vi "Global_CMD_.vi"() -> ()   [LabVIEW 2016]
panel:
  in  "CMD_Subsystem_DBL":dbl
  in  "CMD_Subsystem_Bool":bool
  # "The Names of the Data items in the Global Variable MUST describe who the Single Writer is\nNaming Convention for Command Globals is:   \n\nCMD_SubSystem_Data Name\nExample:\nCMD_Drive_Mode\nCMD_Hopper_Fire Ball"
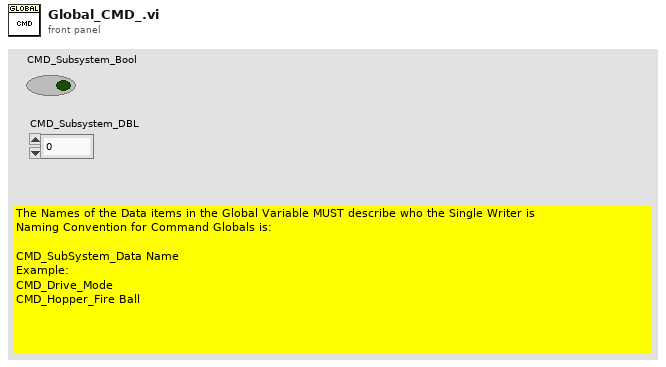
[diagram p1: front panel]
diagram:
